vi "PH_ImageCoG_Plotter.ProcPeriodic.vi"(0 "i ref in":refnum<vi>, 3 "ms timeout (100)":i32=100, 5 "error in (no error)":errorcluster) -> (14 "i ref out":refnum<vi>, 17 "timed out":bool, 19 "error out":errorcluster)   [LabVIEW 2014, in "PH_ImageCoG_Plotter.lvlib"]
doc: "This method serves to periodically do things like reading values from the HW. Methods that should be executed periodically should be called from THIS methode. Add code here."
uses:
  PH_ImageCoG_Plotter.lvlib
  PH_Common/PH_Common.lvlib
  PH_Img_BaseClass/PH_Img_BaseClass.lvlib
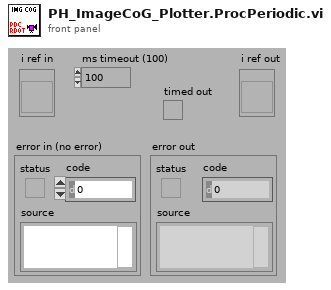
[diagram p1: front panel]
types:
  T1 = typedef "PH_ImageCoG_Plotter.lvlib/PH_ImageCoG_Plotter.i attribute.ctl" = cluster{"GUI Refs":cluster{"Delete":refnum<vi>, "Calibration status":refnum<vi>, "BI subtracted":refnum<vi>, "calc Beam Anal":refnum<vi>, "CoG - x":refnum<vi>, "CoG - y":refnum<vi>, "Type":refnum<vi>, "Center":refnum<vi>, "exp - X":refnum<vi>, "exp - Y":refnum<vi>, "Delta - X":refnum<vi>, "Delta - Y":refnum<vi>, "Available Cams":refnum<vi>, "CoG X":refnum<vi>, "CoG Y":refnum<vi>, "Delta X":refnum<vi>, "Delta Y":refnum<vi>, "Export Data":refnum<vi>, "Calibration data":refnum<vi>}, "Calibration":cluster{"Status":T2, "Calibration data":T3, "Calibration Data File":path}, "Beam Analysis":cluster{"on":bool, "exp - X":i32, "exp - Y":i32, "Type":bool, "Data":cluster{"current time":timestamp, "CoG-x":dbl, "CoG-y":dbl, "Delta-x":dbl, "Delta-y":dbl}[], "Datasets strored":i32, "Dataarray Size":i32}, "Cam instances":string[], "DIM Service Events":T4[], "Images":cluster{"Background":T7, "OP":T7, "GUI":T7}}
  T2 = typedef "PH_StatusHandler.lvlib/PH_StatusHandler.Status.ctl" = i16
  T3 = typedef "PH_ImageCalibrator.lvlib/PH_ImageCalibrator.Calibration Data.ctl" = cluster{"Date":string, "Time":string, "Cam Settings":cluster{"Cam ID":string, "Gain":dbl, "Brightness":dbl, "Shutter":dbl, "Cam Error":bool, "Mode":i32}, "Background Image":cluster{"Image":dbl[][], "Image Error":bool}, "Linear Calibration":cluster{"Calibration Factor":dbl, "not mm or mrad":bool}, "Energy Calibration":cluster{"Calibration Factor":dbl, "no mJ":bool}}
  T4 = typedef "BaseProcess.lvlib/BaseProcess.event definition.ctl" = cluster{"CAEEvtDef":T5, "Data Descriptor":T6}
  T5 = typedef "CAEObj.lvlib/CAEObj.event definition.ctl" = cluster{"URL":string, "enable":bool, "ignoreResID":bool}
  T6 = typedef "BaseProcess.lvlib/BaseProcess.descriptor string definition.ctl" = string
  T7 = typedef "IMAQ Image.ctl" = refnum<image>
  T8 = typedef "PH_Img_BaseClass.lvlib/PH_Img_BaseClass.i attribute.ctl" = cluster{"GUI Refs":T9, "Timeout Image [ms]":i32, "Default Periodic Period [ms]":i32, "Camera":cluster{"Instancename":string, "Notifier":refnum<notifier>}, "Palette":T10, "Cam Settings":cluster{"Cam ID":string, "Gain":dbl, "Brightness":dbl, "Shutter":dbl, "Cam Info Failure":bool, "Mode":i32}}
  T9 = typedef "PH_Img_BaseClass.lvlib/PH_Img_BaseClass.GUI Refs.ctl" = cluster{"Timeout":refnum<vi>, "Image":refnum<vi>, "Palette":refnum<vi>, "Timeout Set":refnum<vi>}
  T10 = typedef "PH_Img_BaseClass.lvlib/PH_Img_BaseClass.Palette.ctl" = i32
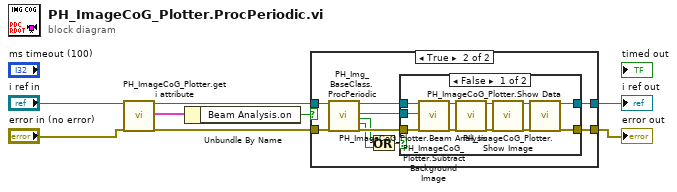
[diagram p0: block diagram]
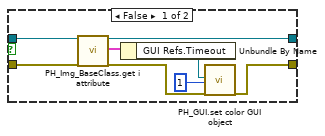
[diagram p2: hidden frame]
diagram:
  n1 = call "PH_ImageCoG_Plotter.get i attribute.vi"("i ref in"="i ref in", "error in (no error)"="error in (no error)") -> ("i ref out"=w4:refnum<vi>, "i attribute"=w8:T1, "error out"=w1:errorcluster)  [unwired: 15 in]
  n2 = Unbundle By Name(w8) -> ("Beam Analysis.on"=w3:bool)
  n3 = case shown="True" w3 {
    tunnel: w4 -> [w12 w26]
    tunnel: w1 -> [w15 w22]
    tunnel: [w14 w24] -> w2
    tunnel: [w11 w25] -> w6
    frame False {
      n4 = call "PH_Img_BaseClass.get i attribute.vi"("i ref in"=w12, "error in (no error)"=w15) -> ("i ref out"=w11:refnum<vi>, "i attribute"=w10:T8, "error out"=w13:errorcluster)  [unwired: 15 in]
      n5 = Unbundle By Name(w10) -> ("GUI Refs.Timeout"=w9:refnum<vi>)
      n6 = call "PH_GUI.set color GUI object.vi"("GUI object Ref"=w9, "State"=1, "error in (no error)"=w13) -> ("error out"=w14:errorcluster)  [unwired: 16 in]
    }
    frame True {
      n7 = call "PH_Img_BaseClass.ProcPeriodic.vi"("i ref in"=w26, "error in (no error)"=w22) -> ("i ref out"=w23:refnum<vi>, "Cam Image"=w20:T7, "timed out?"=w17:bool, "Error while unflatten data?"=w18:bool, "error out"=w21:errorcluster)  [unwired: 13 in]
      n8 = Or(x=w17, y=w18) -> (x .or. y?=w19:bool)
      n9 = case shown="False" w19 {
        tunnel: [w29 w39] -> w25
        tunnel: w21 -> [w37 w38]
        tunnel: w23 -> [w36 w39]
        tunnel: [w28 w38] -> w24
        tunnel: w20 -> [w27 _]
        frame False {
          n10 = call "PH_ImageCoG_Plotter.Subtract Background Image.vi"("i ref in"=w36, "Cam Image"=w27, "error in (no error)"=w37) -> ("i ref out"=w35:refnum<vi>, "error out"=w34:errorcluster)  [unwired: 15 in]
          n11 = call "PH_ImageCoG_Plotter.Beam Analysis.vi"("i ref in"=w35, "error in (no error)"=w34) -> ("i ref out"=w33:refnum<vi>, "error out"=w32:errorcluster)  [unwired: 16 in]
          n12 = call "PH_ImageCoG_Plotter.Show Image.vi"("i ref in"=w33, "error in"=w32) -> ("i ref out"=w31:refnum<vi>, "error out"=w30:errorcluster)  [unwired: 16 in]
          n13 = call "PH_ImageCoG_Plotter.Show Data.vi"("i ref in"=w31, "error in"=w30) -> ("i ref out"=w29:refnum<vi>, "error out"=w28:errorcluster)  [unwired: 16 in]
        }
        frame True {
        }
      }
    }
  }
  "error out" <- w2
  "i ref out" <- w6
